vi "Launch Reusable VI.vi"   [LabVIEW 2020]
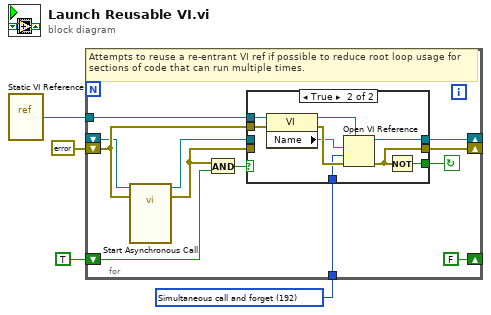
[diagram p0: block diagram]
diagram:
  w3 = 192 items=["Record modifications"=1, "Open templates for editing"=2, "Prompt user to save"=4, "Prepare for reentrant run"=8, "Prompt to find missing subVIs"=16, "Hide loading dialog box"=32, "Enable simultaneous calls"=64, "Prepare to call and forget"=128, "Simultaneous call and forget"=192, "Prepare to call and collect"=256, "Simultaneous call and collect"=320]
  n1 = vi-ref "Static VI Reference"() -> ("vi reference"=w4:refnum<vi>)
  n2 = for {
    tunnel: w4 -> [w15]
    tunnel: w3 -> [w14]
    shift-right: [w13] -> _
    shift-left: _ -> [w12]
    shift-right: [w10] -> _
    shift-left: errorcluster {"status"=FALSE, "code"=0, "source"=""} ("error constant") -> [w16]
    shift-right: [FALSE] -> _
    shift-left: TRUE -> [w7]
    stop <- w6 continue-if-true
    # "Attempts to reuse a re-entrant VI ref if possible to reduce root loop usage for sections of code that can run multiple times."
    n3 = call-by-ref "Start Asynchronous Call"(reference=w12, error in=w16) -> (reference out=w11:refnum<vi>, error out=w9:errorcluster)
    n4 = And(x=w9, y=w7) -> (x .and. y?=w8:bool)
    n5 = case shown="True" w8 {
      tunnel: w15 -> [_ w26]
      tunnel: w14 -> [_ w24]
      tunnel: [w18 w22] -> w13
      tunnel: w11 -> [w18 _]
      tunnel: [w17 w20] -> w10
      tunnel: w9 -> [w17 _]
      tunnel: w16 -> [_ w21]
      tunnel: [_ w19] -> w6
      frame False {
      }
      frame True {
        n6 = property class="VI"(reference=w26, error in=w21) -> (reference out=w23:refnum<vi>, error out=w27:errorcluster, "Name"=w25:string)
        n7 = Open VI Reference(type specifier VI Refnum (for type only)=w23, vi path=w25, options=w24, error in (no error)=w27) -> (vi reference=w22:refnum<vi>, error out=w20:errorcluster)  [unwired: 2 in]
        n8 = Not(x=w20) -> (.not. x?=w19:bool)
      }
    }
  }
